vi "SRDG535.ProcPeriodic.vi"(0 "i ref in":refnum<vi>, 3 "ms timeout (100)":i32=100, 5 "error in (no error)":errorcluster) -> (14 "i ref out":refnum<vi>, 17 "timed out":bool, 19 "error out":errorcluster)   [LabVIEW 2014, in "SRDG535.lvlib"]
doc: "This method serves to periodically do things like reading values from the HW. Methods that should be executed periodically should be called from THIS methode. Add code here."
uses:
  SRDG535.lvlib
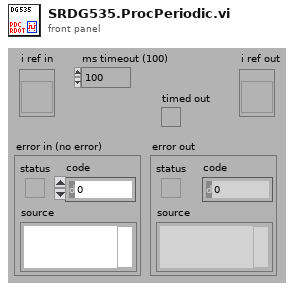
[diagram p1: front panel]
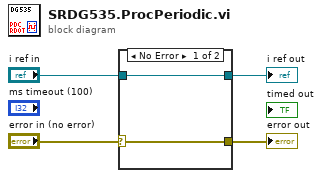
[diagram p0: block diagram]
diagram:
  n1 = case shown="No Error" "error in (no error)" {
    selector: "error in (no error)" -> [w6 w8]
    tunnel: [w6 w8] -> w3
    tunnel: "i ref in" -> [w5 w7]
    tunnel: [w5 w7] -> w1
    frame No Error {
    }
    frame Error {
    }
  }
  "error out" <- w3
  "i ref out" <- w1
